vi "Level.vi"(3 "Y_Lev_max":dbl=80.0 format="%#_13g", 4 "IN":dbl=20.0, 5 "G_Lev_max":dbl=30.0 format="%#_13g") -> (0 "R":bool, 1 "Y":bool, 2 "G":bool)   [LabVIEW 2018]
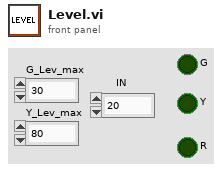
[diagram p1: front panel]
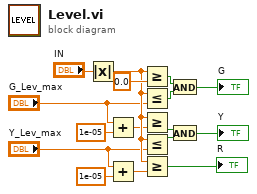
[diagram p0: block diagram]
diagram:
  n1 = Absolute Value(x="IN") -> (abs(x)=w11:dbl)
  n2 = Add(x="G_Lev_max", y=1e-05) -> (x+y=w6:dbl)
  n3 = Add(x="Y_Lev_max", y=1e-05) -> (x+y=w1:dbl)
  n4 = Greater Or Equal?(x=w11, y=0.0) -> (x >= y?=w14:bool)
  n5 = Less Or Equal?(x=w11, y="G_Lev_max") -> (x <= y?=w15:bool)
  n6 = Greater Or Equal?(x=w11, y=w6) -> (x >= y?=w12:bool)
  n7 = Less Or Equal?(x=w11, y="Y_Lev_max") -> (x <= y?=w13:bool)
  n8 = Greater Or Equal?(x=w11, y=w1) -> (x >= y?=→"R":bool)
  n9 = And(x=w14, y=w15) -> (x .and. y?=→"G":bool)
  n10 = And(x=w12, y=w13) -> (x .and. y?=→"Y":bool)
